vi "LED-New Text.vi"(11 "Current Text":string) -> (2 "New text":string, 3 "Cancelled?":bool)   [LabVIEW 2010, in "LED Display.xctl"]
doc: "Use this template to create a dialog box with event handling."
uses:
  LED Display.xctl
panel:
  in  "Enter new text...":string
  in  "Cancel":bool
  in  "OK":bool
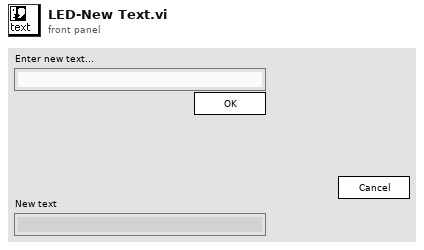
[diagram p1: front panel]
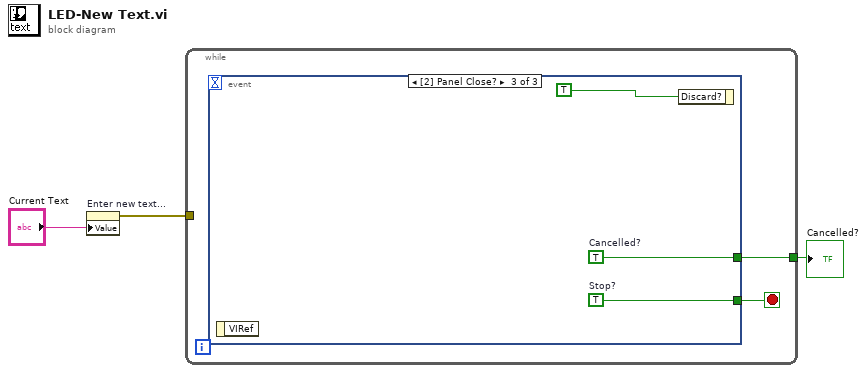
[diagram p0: block diagram]
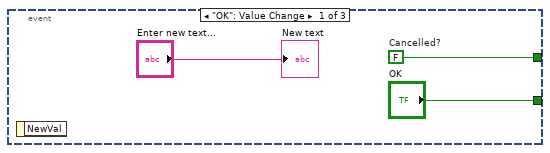
[diagram p2: hidden frame]
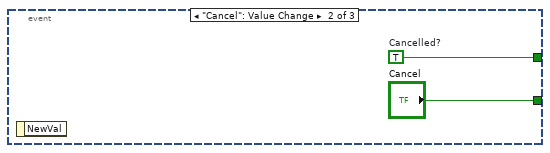
[diagram p3: hidden frame]
diagram:
  n1 = property on="Enter new text..." class="Str"("Value"="Current Text") -> (error out=w1:errorcluster)  [unwired: 2 in, 1 out]
  n2 = while {
    tunnel: [w4] -> w3
    tunnel: w1 -> [_]
    stop <- w5 stop-if-true
    n3 = event shown="[2] Panel Close?" {
      selector: _ -> [_ _ _]
      dyn-events: _ -> [_ _ _]
      timeout: _ -> [_ _ _]
      tunnel: ["OK" "Cancel" w12] -> w5
      tunnel: [w8 w10 w11] -> w4
      event "OK": Value Change {
        w8 = FALSE  # Cancelled?
        n4 = event-data() -> ()  [unwired: 1 in, 1 out]
        "New text" <- "Enter new text..."
      }
      event "Cancel": Value Change {
        w10 = TRUE  # Cancelled?
        n5 = event-data() -> ()  [unwired: 1 in, 1 out]
      }
      event Panel Close? {
        w11 = TRUE  # Cancelled?
        w12 = TRUE  # Stop?
        n6 = event-data() -> ()  [unwired: 1 in, 1 out]
        n7 = event-data("Discard?"=TRUE) -> ()  [unwired: 1 in, 1 out]
      }
    }
  }
  "Cancelled?" <- w3
